vi "Omni Odometry.vi"(9 "dt":dbl, 10 "TaimiOmniVelocity":T3, 11 "OmniDynamics in":T1={"frame_id"="", "child_frame_id"="", "PoseCovariance"={"Pose"={"Point"={"x"=0.0, "y"=0.0, "z"=0.0}, "Quaternion"={"x"=0.0, "y"=0.0, "z"=0.0, "w"=0.0}}, "Covariance"=[0.0, 0.0, 0.0, 0.0, 0.0]}, "TwistCovariance"={"Twist"={"Linear"={"x"=0.0, "y"=0.0, "z"=0.0}, "Angular"={"x"=0.0, "y"=0.0, "z"=0.0}}, "Covariance"=[0.0, 0.0, 0.0, 0.0, 0.0]}}) -> (3 "OmniDynamics out":T1)   [LabVIEW 2014]
uses:
  <vilib>/robotics/TaimiOmni/TaimiOmni/TaimiOmniVelocity.ctl
  Odometry.ctl
  TwistCovariance.ctl
  <vilib>/Analysis/baseanly.llb/A x Vector.vi
  <vilib>/Analysis/baseanly.llb/Outer Product.vi
  <vilib>/Analysis/baseanly.llb/Real Outer Product.vi
  <vilib>/robotics/Kinematics/Create Lie Group Matrix.vi
  <vilib>/robotics/Kinematics/RotateX.vi
  <vilib>/robotics/Kinematics/RotateY.vi
  <vilib>/robotics/Kinematics/RotateZ.vi
  <vilib>/Analysis/baseanly.llb/Real A x B.vi
  <vilib>/Analysis/Matrix/Numeric/Multiply/Multiply.vi
  <vilib>/Analysis/Matrix/Numeric/Multiply/Multiply - RM,R.vi
  <vilib>/Analysis/Matrix/Numeric/Multiply/Multiply - R,RM.vi
  <vilib>/Analysis/Matrix/Numeric/Add/Add.vi
  <vilib>/Analysis/Matrix/Numeric/Add/Add - RM,RM.vi
  <vilib>/robotics/Kinematics/Rotation Matrix to Angle Vector.vi
  <vilib>/robotics/Kinematics/NI_Kinematics.lvlib
  <vilib>/Analysis/NI_AALBase.lvlib
  <vilib>/robotics/TaimiOmni/TaimiOmni/TaimiOmni.lvclass
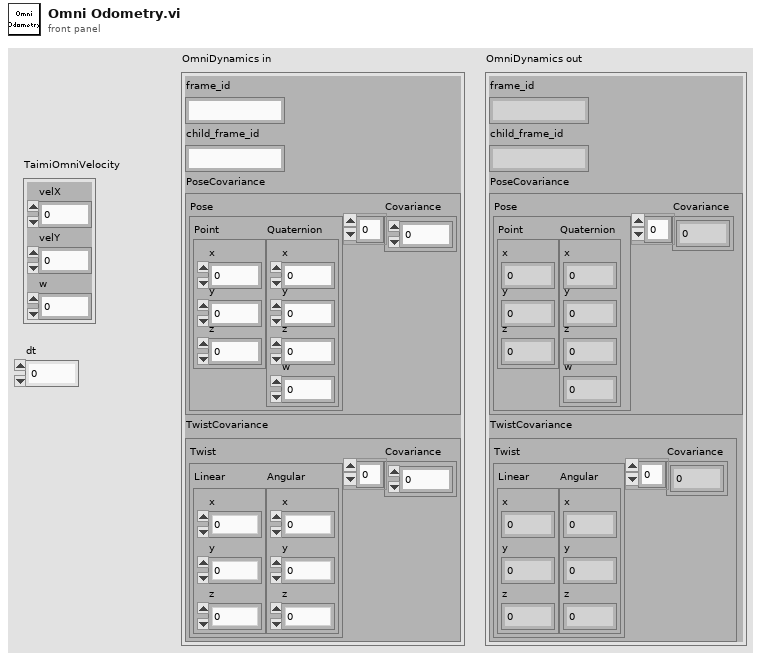
[diagram p1: front panel]
types:
  T1 = typedef "Odometry.ctl" = cluster{"frame_id":string, "child_frame_id":string, "PoseCovariance":cluster{"Pose":cluster{"Point":cluster{"x":dbl, "y":dbl, "z":dbl}, "Quaternion":cluster{"x":dbl, "y":dbl, "z":dbl, "w":dbl}}, "Covariance":dbl[]}, "TwistCovariance":T2}
  T2 = typedef "TwistCovariance.ctl" = cluster{"Twist":cluster{"Linear":cluster{"x":dbl, "y":dbl, "z":dbl}, "Angular":cluster{"x":dbl, "y":dbl, "z":dbl}}, "Covariance":dbl[]}
  T3 = typedef "TaimiOmni.lvclass/TaimiOmniVelocity.ctl" = cluster{"velX":dbl, "velY":dbl, "w":dbl}
  T4 = typedef "NI_Matrix.lvlib/RealMatrix.ctl" = dbl[][]
  T5 = typedef "NI_Kinematics.lvlib/Quaternion.ctl" = dbl[]
  T6 = cluster{"Numeric":dbl, "Numeric":dbl, "Numeric":dbl, "Numeric":dbl}
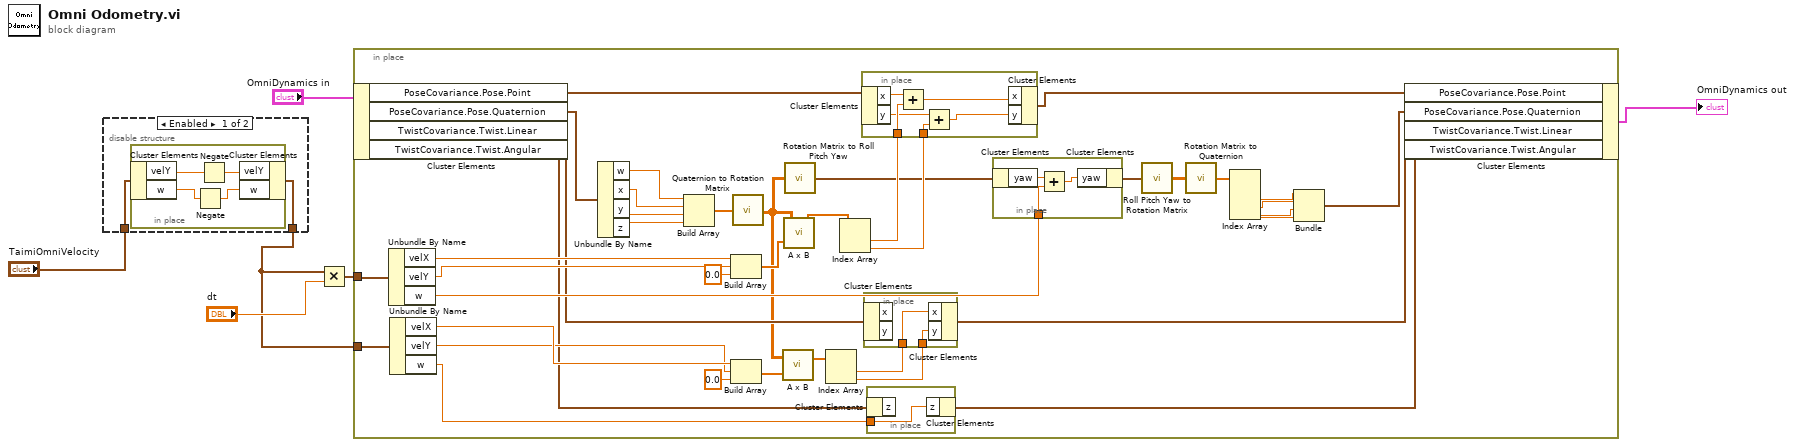
[diagram p0: block diagram]
diagram:
  n1 = disable-structure shown="Enabled" {
    disable-tunnel: "TaimiOmniVelocity" -> [w8 w13]
    disable-tunnel: [w7 w13] -> w1
    frame Enabled {
      n2 = in-place {
        n3 = in-place-cluster #1(w8) -> ("velY"=w12:dbl, "w"=w9:dbl)
        n4 = Negate(x=w9) -> (-x=w10:dbl)
        n5 = Negate(x=w12) -> (-x=w11:dbl)
        n6 = in-place-cluster #1("velY"=w11, "w"=w10) -> (w7:T3)
      }
    }
    frame Disabled {
    }
  }
  n7 = Multiply(x=w1, y="dt") -> (x*y=w3:T3)
  n8 = in-place {
    in-place-border: w3 -> [w53]
    in-place-border: w1 -> [w39]
    n9 = in-place-cluster #2("OmniDynamics in") -> ("PoseCovariance.Pose.Point"=w52:cluster{"x":dbl, "y":dbl, "z":dbl}, "PoseCovariance.Pose.Quaternion"=w25:cluster{"x":dbl, "y":dbl, "z":dbl, "w":dbl}, "TwistCovariance.Twist.Linear"=w38:cluster{"x":dbl, "y":dbl, "z":dbl}, "TwistCovariance.Twist.Angular"=w28:cluster{"x":dbl, "y":dbl, "z":dbl})
    n10 = Unbundle By Name(w53) -> ("velX"=w51:dbl, "velY"=w50:dbl, "w"=w43:dbl)
    n11 = Unbundle By Name(w39) -> ("velX"=w36:dbl, "velY"=w35:dbl, "w"=w27:dbl)
    n12 = Unbundle By Name(w25) -> ("w"=w24:dbl, "x"=w23:dbl, "y"=w22:dbl, "z"=w21:dbl)
    n13 = Build Array(w24, w23, w22, w21) -> (w20:dbl[])
    n14 = Build Array(w51, w50, 0.0 ("element")) -> (w48:dbl[])
    n15 = Build Array(w36, w35, 0.0 ("element")) -> (w33:dbl[])
    n16 = call <vilib>:"Quaternion to Rotation Matrix.vi"("quaternion"=w20) -> ("rotation matrix"=w34:T4)
    n17 = call-poly <vilib>:"A x B.vi"("Vector"=w33, "A"=w34) -> ("A x Vector"=w32:dbl[])  [unwired: 1 out]
    n18 = call-poly <vilib>:"A x B.vi"("Vector"=w48, "A"=w34) -> ("A x Vector"=w47:dbl[])  [unwired: 1 out]
    n19 = call <vilib>:"Rotation Matrix to Roll Pitch Yaw.vi"("rotation matrix"=w34) -> ("angles"=w44:cluster{"roll":dbl, "pitch":dbl, "yaw":dbl})
    n20 = Index Array(array=w32) -> (element #1=w31:dbl, element #2=w30:dbl)  [unwired: 2 in]
    n21 = Index Array(array=w47) -> (element #1=w46:dbl, element #2=w45:dbl)  [unwired: 2 in]
    n22 = in-place {
      in-place-border: w46 -> [w64]
      in-place-border: w45 -> [w61]
      n23 = in-place-cluster #3(w52) -> ("x"=w65:dbl, "y"=w62:dbl)
      n24 = Add(x=w65, y=w64) -> (x+y=w63:dbl)
      n25 = Add(x=w62, y=w61) -> (x+y=w60:dbl)
      n26 = in-place-cluster #3("x"=w63, "y"=w60) -> (w40:cluster{"x":dbl, "y":dbl, "z":dbl})
    }
    n27 = in-place {
      in-place-border: w31 -> [w56]
      in-place-border: w30 -> [w55]
      n28 = in-place-cluster #4(w38) -> ()  [unwired: 2 out]
      n29 = in-place-cluster #4("x"=w56, "y"=w55) -> (w29:cluster{"x":dbl, "y":dbl, "z":dbl})
    }
    n30 = in-place {
      in-place-border: w27 -> [w54]
      n31 = in-place-cluster #5(w28) -> ()  [unwired: 1 out]
      n32 = in-place-cluster #5("z"=w54) -> (w26:cluster{"x":dbl, "y":dbl, "z":dbl})
    }
    n33 = in-place {
      in-place-border: w43 -> [w58]
      n34 = in-place-cluster #6(w44) -> ("yaw"=w59:dbl)
      n35 = Add(x=w59, y=w58) -> (x+y=w57:dbl)
      n36 = in-place-cluster #6("yaw"=w57) -> (w42:cluster{"roll":dbl, "pitch":dbl, "yaw":dbl})
    }
    n37 = call <vilib>:"Roll Pitch Yaw to Rotation Matrix.vi"("angles"=w42) -> ("rotation matrix"=w41:T4)
    n38 = call <vilib>:"Rotation Matrix to Quaternion.vi"("rotation matrix"=w41) -> ("quaternion"=w19:T5)
    n39 = Index Array(array=w19) -> (element #1=w15:dbl, element #2=w18:dbl, element #3=w17:dbl, element #4=w16:dbl)  [unwired: 4 in]
    n40 = Bundle("Numeric"=w18, "Numeric"=w17, "Numeric"=w16, "Numeric"=w15) -> (w14:T6)  [unwired: 1 in]
    n41 = in-place-cluster #2("PoseCovariance.Pose.Point"=w40, "PoseCovariance.Pose.Quaternion"=w14, "TwistCovariance.Twist.Linear"=w29, "TwistCovariance.Twist.Angular"=w26) -> (→"OmniDynamics out":T1)
  }
